vi "Welcome UI _ Read System Logo and title.vi"(8 "error in":errorcluster caption="错误输入", 10 "file folder in":path, 11 "file in":path) -> (0 "error out":errorcluster caption="错误输出", 2 "para out":T1)   [LabVIEW 2016]
uses:
  <vilib>/Utility/config.llb/Read Key (String).vi
  Ctrls/GlobeVaribles.vi
  <vilib>/Utility/config.llb/NI_LVConfig.lvlib
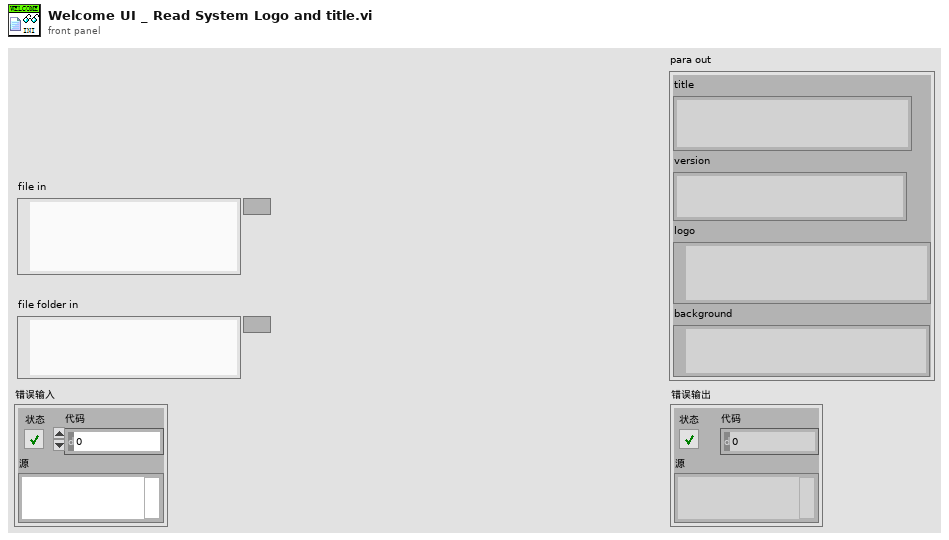
[diagram p1: front panel]
types:
  T1 = cluster{"title":string, "version":string, "logo":path, "background":path}
  T2 = typedef "NI_LVConfig.lvlib/Config Data RefNum.ctl" = refnum<k1>
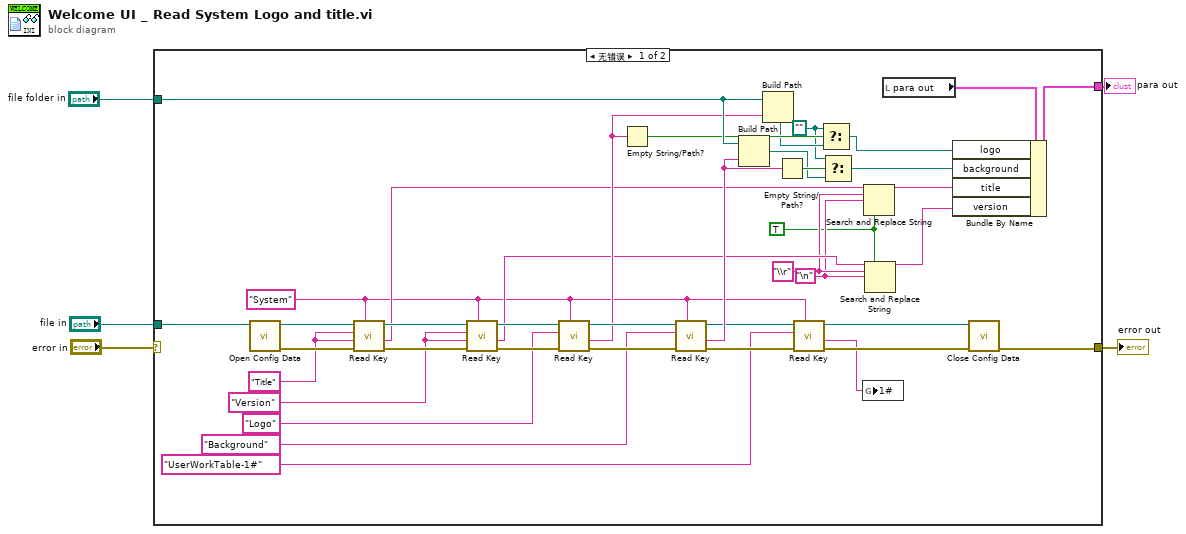
[diagram p0: block diagram]
diagram:
  n1 = case shown="无错误" "error in" {
    selector: "error in" -> [_ w46]
    tunnel: [w30 w46] -> w4
    tunnel: "file in" -> [w45 _]
    tunnel: "file folder in" -> [w31 _]
    tunnel: [w29 _] -> w1
    frame No Error {
      w14 = "\n"
      w15 = "\\r" ("搜索字符串")
      w13 = TRUE ("替换全部？(F)")
      w24 = path ""
      w35 = "Version" ("section")
      w36 = "Title" ("section")
      w8 = "System" ("section")
      n2 = call <vilib>:"Open Config Data.vi"("configuration file path"=w45) -> ("error out"=w44:errorcluster, "refnum"=w43:T2)  [unwired: 8 in, 1 out]
      n3 = call-poly <vilib>:"Read Key.vi"("section"=w8, "error in (no error)"=w44, "default value"=w36, "key"=w36, "refnum"=w43) -> ("error out"=w42:errorcluster, "value"=w17:string, "refnum out"=w41:T2)  [unwired: 3 in, 1 out]
      n4 = call-poly <vilib>:"Read Key.vi"("section"=w8, "error in (no error)"=w42, "default value"=w35, "key"=w35, "refnum"=w41) -> ("error out"=w37:errorcluster, "value"=w18:string, "refnum out"=w40:T2)  [unwired: 3 in, 1 out]
      n5 = call-poly <vilib>:"Read Key.vi"("section"=w8, "error in (no error)"=w37, "key"="Logo" ("section"), "refnum"=w40) -> ("error out"=w38:errorcluster, "value"=w28:string, "refnum out"=w39:T2)  [unwired: 4 in, 1 out]
      n6 = Empty String/Path?(string/path=w28) -> (empty?=w27:bool)
      n7 = call-poly <vilib>:"Read Key.vi"("section"=w8, "error in (no error)"=w38, "key"="Background" ("section"), "refnum"=w39) -> ("error out"=w11:errorcluster, "value"=w23:string, "refnum out"=w12:T2)  [unwired: 4 in, 1 out]
      n8 = Build Path(base path=w31, name or relative path=w23) -> (appended path=w21:path)
      n9 = Build Path(base path=w31, name or relative path=w28) -> (appended path=w26:path)
      n10 = Empty String/Path?(string/path=w23) -> (empty?=w22:bool)
      n11 = call-poly <vilib>:"Read Key.vi"("section"=w8, "error in (no error)"=w11, "key"="UserWorkTable-1#" ("section"), "refnum"=w12) -> ("error out"=w10:errorcluster, "value"=w6:string, "refnum out"=w9:T2)  [unwired: 4 in, 1 out]
      n12 = Select(t=w24, s=w27, f=w26) -> (s? t:f=w25:path)
      n13 = Select(t=w24, s=w22, f=w21) -> (s? t:f=w20:path)
      n14 = global write "GlobeVaribles.vi" "1#"(w6) -> ()
      n15 = Search and Replace String(replace all?=w13, input string=w17, search string=w15, replace string=w14) -> (result string=w16:string)  [unwired: 4 in, 3 out]
      n16 = Search and Replace String(replace all?=w13, input string=w18, search string=w15, replace string=w14) -> (result string=w19:string)  [unwired: 4 in, 3 out]
      n17 = local read "para out"() -> (w32:T1)
      n18 = Bundle By Name(cluster=w32, "logo"=w25, "background"=w20, "title"=w16, "version"=w19) -> (w29:T1)
      n19 = call <vilib>:"Close Config Data.vi"("error in (no error)"=w10, "refnum"=w9) -> ("error out"=w30:errorcluster)  [unwired: 8 in, 1 out]
    }
    frame Error {
    }
  }
  "error out" <- w4
  "para out" <- w1
